vi "GPIB_findInstrument.vi"(9 "ID command":string, 10 "revised GPIB address":string, 11 "Instrument name IN":string) -> (2 "revised GPIB address OUT":string)   [LabVIEW 2019, in "InstrControl.lvclass"]
uses:
  InstrControl.lvclass
panel:
  in  "Refresh Button":bool
  in  "Cancel":bool
  in  "OK":bool
  out "instrument responses":string[](array[string])
  out "instrument addresses found":string[](array[string])
  out "error out":errorcluster
  in  "error in (no error)":errorcluster
  # "Find GPIB instrument:"
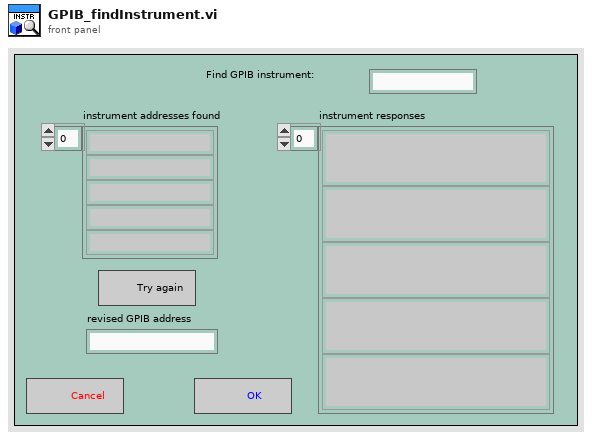
[diagram p1: front panel]
types:
  T1 = cluster{"error":bool, "code":i32, "source":string}
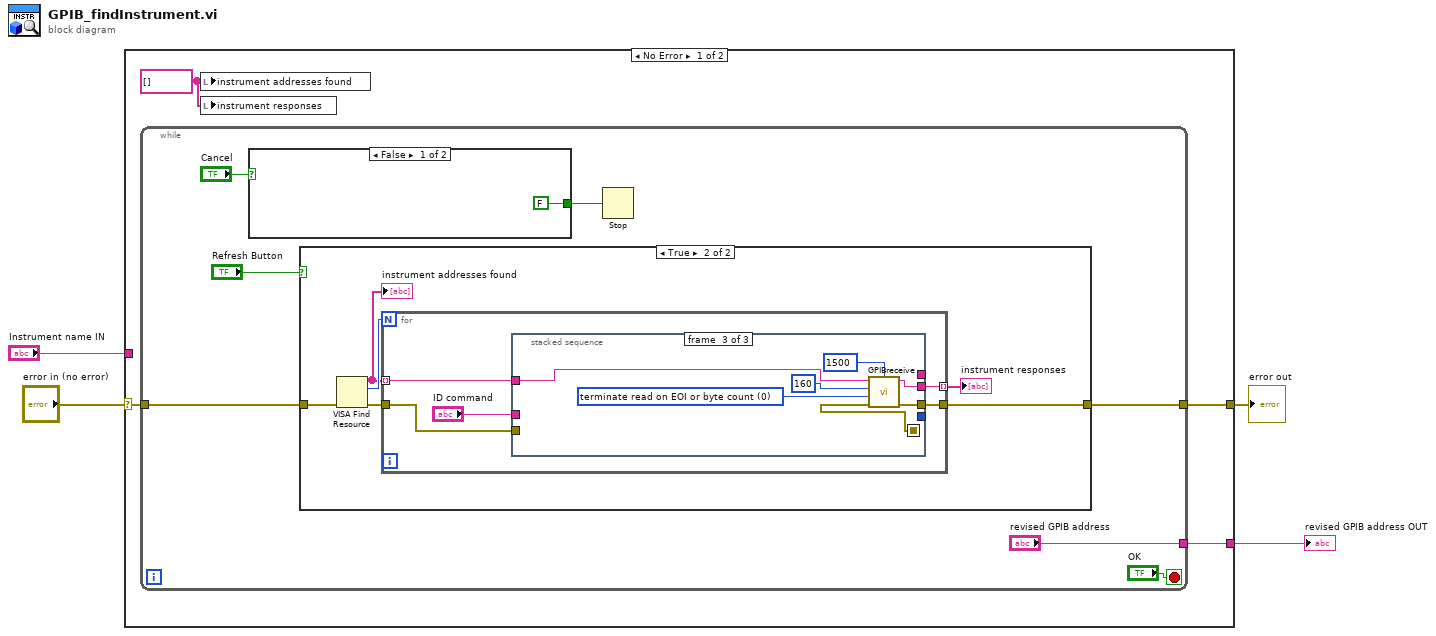
[diagram p0: block diagram]
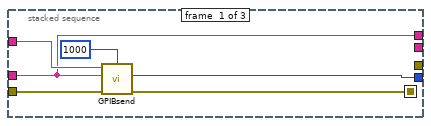
[diagram p3: hidden frame]
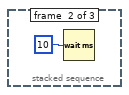
[diagram p4: hidden frame]
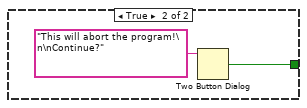
[diagram p5: hidden frame]
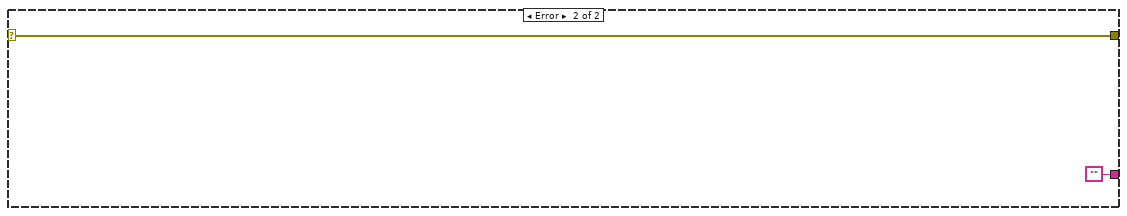
[diagram p6: hidden frame]
diagram:
  n1 = case shown="No Error" "error in (no error)" {
    selector: "error in (no error)" -> [w8 w46]
    tunnel: [w7 w46] -> w3
    tunnel: [w6 ""] -> w2
    tunnel: "Instrument name IN" -> [_ _]
    frame No Error {
      w5 = string[] []
      n2 = while {
        tunnel: w8 -> [w15]
        tunnel: [w11] -> w7
        tunnel: ["revised GPIB address"] -> w6
        stop <- "OK" stop-if-true
        n3 = case shown="False" "Cancel" {
          tunnel: [FALSE w43] -> w13
          frame False {
          }
          frame True {
            n4 = Two Button Dialog(message="This will abort the program!\n\nContinue?") -> (T button?=w43:bool)  [unwired: 2 in]
          }
        }
        n5 = case shown="True" "Refresh Button" {
          tunnel: w15 -> [w16 w20]
          tunnel: [w16 w17] -> w11
          frame False {
          }
          frame True {
            n6 = VISA Find Resource(8:w20) -> (0:w22:errorcluster, 2:w21:u32, 3:w19:string[])  [unwired: 2 in]
            "instrument addresses found" <- w19
            n7 = for {
              N: w21 -> [_]
              tunnel: w19 -> [w24] mode=indexing
              tunnel: w22 -> [w27]
              tunnel: [w26] -> w17
              tunnel: [w25] -> w18 mode=indexing
              n8 = stacked-sequence {
                seq-local: [w31 _ _] -> [_ _ w40]
                tunnel: w24 -> [w33 _ w39]
                tunnel: w27 -> [w32 _ _]
                tunnel: [_ _ w41] -> w26
                tunnel: [w29 _ _] -> _
                tunnel: [_ _ w37] -> w25
                tunnel: "ID command" -> [w29 _ _]
                tunnel: [w28 _ _] -> _
                frame #0 {
                  n9 = call "GPIBsend.vi"("timeout ms"=u32 1000, "address string"=w33, "write buffer"=w29, "error in"=w32) -> ("byte count"=w28:i32, "error out"=w31:errorcluster)  [unwired: 3 in, 1 out]
                }
                frame #1 {
                  n10 = Wait (ms)(milliseconds to wait=10) -> ()  [unwired: 1 out]
                }
                frame #2 {
                  w36 = 0 items=["terminate read on EOI or byte count", "terminate read on EOI, byte count, or CR", "terminate read on EOI, byte count, or LF"] ("read mode")
                  n11 = call "GPIBreceive.vi"("timeout ms"=u32 1500, "address string"=w39, "byte count"=160, "read mode"=w36, "error in"=w40) -> ("read buffer"=w37:string, "error out"=w41:T1)  [unwired: 2 in, 1 out]
                }
              }
            }
            "instrument responses" <- w18
          }
        }
        n12 = Stop(stop? (T)=w13) -> ()
      }
      n13 = local write "instrument addresses found"(w5) -> ()
      n14 = local write "instrument responses"(w5) -> ()
    }
    frame Error {
    }
  }
  "error out" <- w3
  "revised GPIB address OUT" <- w2
